vi "Works slow.vi"() -> ()   [LabVIEW 2024]
panel:
  in  "stop":bool
  out "return value":dbl[](array[numeric])
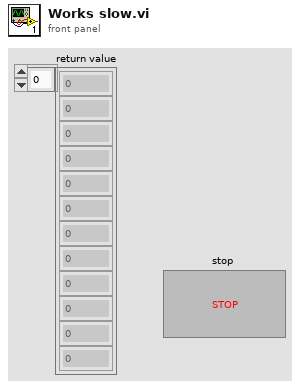
[diagram p1: front panel]
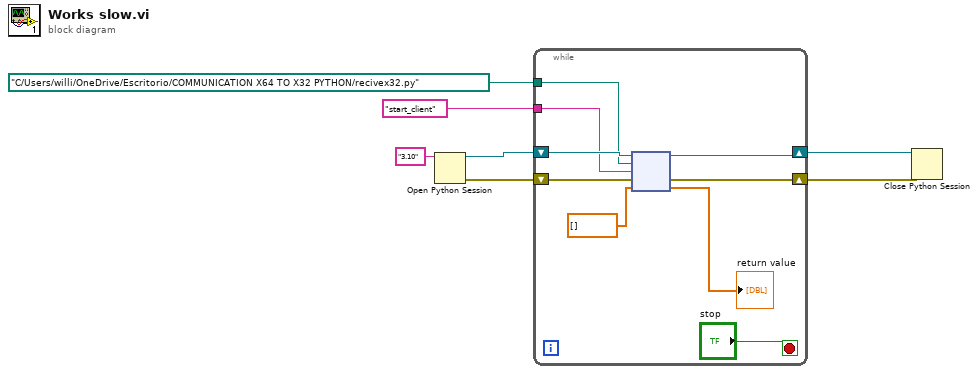
[diagram p0: block diagram]
diagram:
  n1 = Open Python Session(python version="3.10" ("Python version")) -> (session out=w7:refnum<k35>, error out=w4:errorcluster)  [unwired: 2 in]
  n2 = while {
    tunnel: path "C:/Users/willi/OneDrive/Escritorio/COMMUNICATION X64 TO X32 PYTHON/recivex32.py" ("module path") -> [w12]
    tunnel: "start_client" ("function name") -> [w11]
    shift-right: [w15] -> w6
    shift-left: w7 -> [w16]
    shift-right: [w14] -> w5
    shift-left: w4 -> [w13]
    stop <- "stop" stop-if-true
    n3 = node(w16, w12, w11, w13, dbl[] []) -> (w15:refnum<k35>, w14:errorcluster, →"return value":dbl[])  [unwired: 2 out]
  }
  n4 = Close Python Session(session in=w6, error in=w5) -> ()  [unwired: 1 out]
